vi "Aula 4 24_08 cluster_tunnel.vi"() -> ()   [LabVIEW 2020]
panel:
  out "Waveform Chart":dbl(graph)
  out "Ângulo-1":dbl
  out "Último":dbl
  out "Valor aleatório (0-1)":dbl
  out "Ângulo[º]":dbl
  out "Ângulo [rad]":dbl
  out "Função":cluster{dbl, dbl, "number: 0 to 1":dbl}(graph)
  in  "Segundos":dbl
  in  "Stop":bool
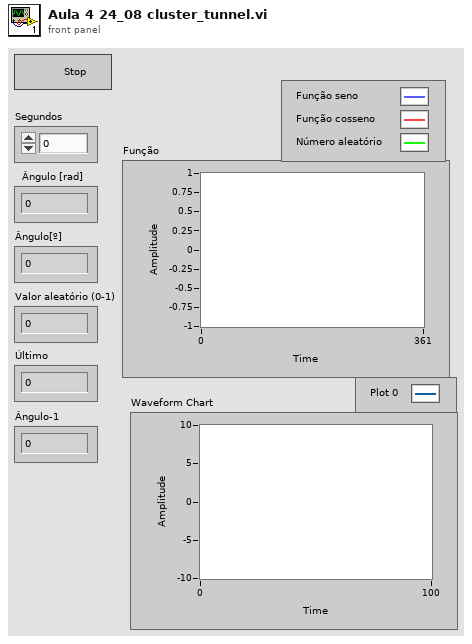
[diagram p1: front panel]
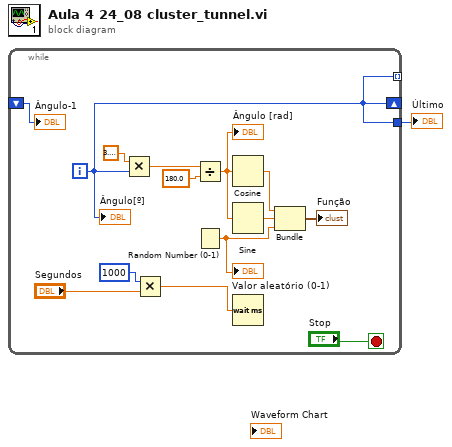
[diagram p0: block diagram]
diagram:
  n1 = while {
    tunnel: [w2] -> w1
    shift-right: [w2] -> _
    shift-left: _ -> [w3]
    tunnel: [w2] -> _ mode=indexing
    i -> [w2]
    stop <- "Stop" stop-if-true
    n2 = Multiply(x=3.141592653589793, y=w2) -> (x*y=w10:dbl)
    n3 = Multiply(x=u32 1000 ("x*y"), y="Segundos") -> (x*y=w12:dbl)
    n4 = Divide(x=w10, y=180.0 ("x")) -> (x/y=w8:dbl)
    "Ângulo [rad]" <- w8
    n5 = Random Number (0-1)() -> (number: 0 to 1=w4:dbl)
    "Valor aleatório (0-1)" <- w4
    n6 = Cosine(x=w8) -> (cos(x)=w6:dbl)
    n7 = Sine(x=w8) -> (sin(x)=w7:dbl)
    n8 = Wait (ms)(milliseconds to wait=w12) -> ()  [unwired: 1 out]
    n9 = Bundle(w6, w7, "number: 0 to 1"=w4) -> (→"Função":cluster{dbl, dbl, "number: 0 to 1":dbl})  [unwired: 1 in]
    "Ângulo[º]" <- w2
    "Ângulo-1" <- w3
  }
  "Último" <- w1
